vi "GraspMapTHIN.vi"(1 "copyIN (m)":dbl, 2 "copxIN (m)":dbl, 3 "copyTH (m)":dbl=0.0216, 4 "copxTH (m)":dbl=0.0216) -> (0 "Grasp Map":T1)   [LabVIEW 2021]
uses:
  <vilib>/Analysis/Matrix/Datatypes/RealMatrix.ctl
  <vilib>/Analysis/baseanly.llb/Real A x B.vi
  <vilib>/Analysis/Matrix/NI_Matrix.lvlib
  <vilib>/Analysis/NI_AALBase.lvlib
panel:
  in  "half handle width (m)":dbl=0.0216
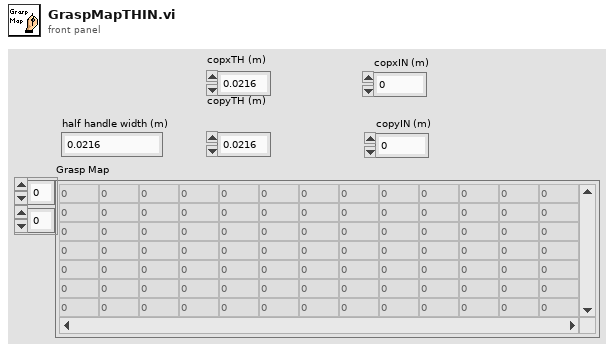
[diagram p1: front panel]
types:
  T1 = typedef "NI_Matrix.lvlib/RealMatrix.ctl" = dbl[][]
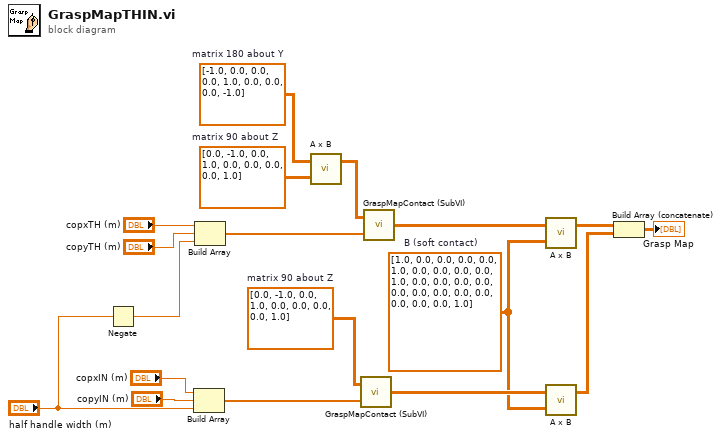
[diagram p0: block diagram]
diagram:
  w2 = T1 [[1.0, 0.0, 0.0, 0.0], [0.0, 1.0, 0.0, 0.0], [0.0, 0.0, 1.0, 0.0], [0.0, 0.0, 0.0, 0.0], [0.0, 0.0, 0.0, 0.0], [0.0, 0.0, 0.0, 1.0]]  # B (soft contact)
  w15 = T1 [[0.0, -1.0, 0.0], [1.0, 0.0, 0.0], [0.0, 0.0, 1.0]]  # matrix 90 about Z
  w16 = T1 [[0.0, -1.0, 0.0], [1.0, 0.0, 0.0], [0.0, 0.0, 1.0]]  # matrix 90 about Z
  w14 = T1 [[-1.0, 0.0, 0.0], [0.0, 1.0, 0.0], [0.0, 0.0, -1.0]]  # matrix 180 about Y
  n1 = Negate(x="half handle width (m)") -> (-x=w11:dbl)
  n2 = Build Array("copxIN (m)", "copyIN (m)", "half handle width (m)") -> (w6:dbl[])
  n3 = Build Array("copxTH (m)", "copyTH (m)", w11) -> (w10:dbl[])
  n4 = call-poly <vilib>:"A x B.vi"("B"=w16, "A"=w14) -> ("A x B"=w17:T1)  [unwired: 1 out]
  n5 = call "GraspMapContact (SubVI).vi"("position Vector"=w6, "r matrix"=w15) -> ("contact grasp map matrix"=w3:T1)
  n6 = call "GraspMapContact (SubVI).vi"("position Vector"=w10, "r matrix"=w17) -> ("contact grasp map matrix"=w4:T1)
  n7 = call-poly <vilib>:"A x B.vi"("B"=w2, "A"=w4) -> ("A x B"=w5:T1)  [unwired: 1 out]
  n8 = call-poly <vilib>:"A x B.vi"("B"=w2, "A"=w3) -> ("A x B"=w1:T1)  [unwired: 1 out]
  n9 = Build Array (concatenate) ("Build Matrix")(w5, w1) -> (→"Grasp Map":T1)
